vi "LVIS_Test.vi"(8 "Error In":errorcluster, 11 "TestInfo":T1) -> (0 "Error Out":errorcluster)   [LabVIEW 2015]
doc: "Determines the Test Info based on the LVIS_Settings file and passed in values, giving precedence to the file and deriving values where requested. Validates all test data."
uses:
  Sub VIs/Globals/LVIS_IsGlobal.vi
panel:
  out "DateTime":string
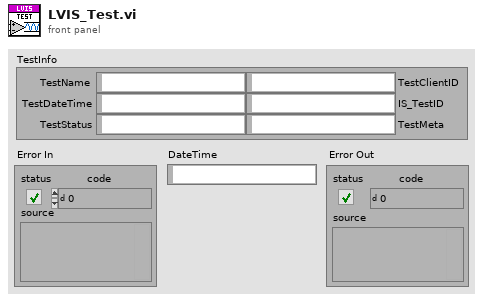
[diagram p1: front panel]
types:
  T1 = cluster{"TestName":string, "TestDateTime":string, "TestStatus":string, "TestClientID":string, "IS_TestID":string, "TestMeta":string}
  T2 = cluster{"[0]":string, "[1]":string, "[2]":string, "[3]":string, "[4]":string, "[5]":string}
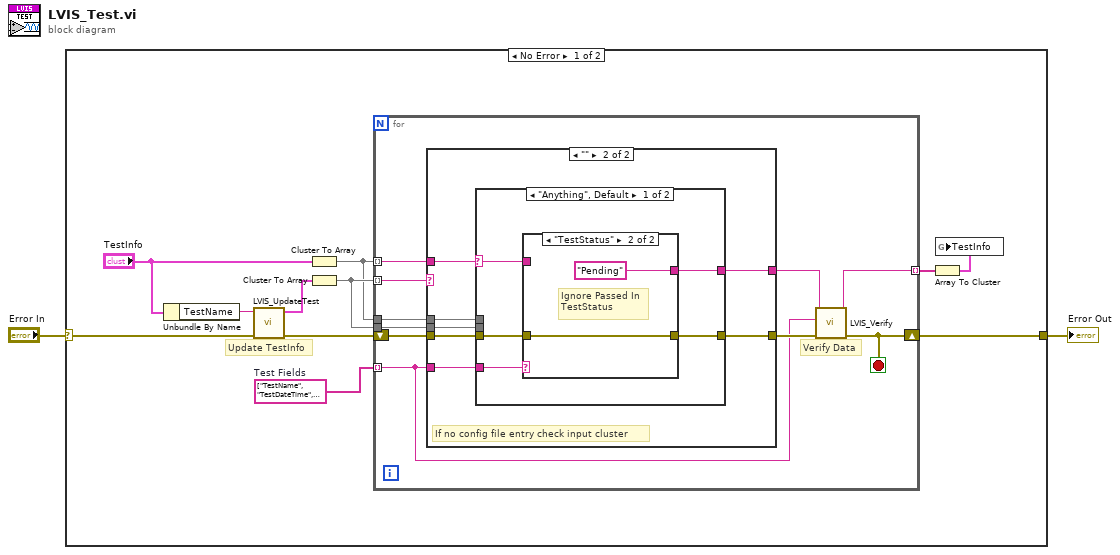
[diagram p0: block diagram]
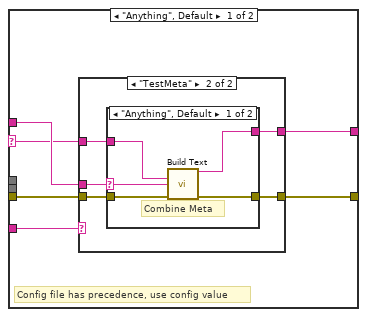
[diagram p2: hidden frame]
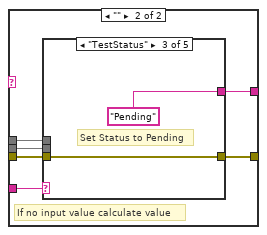
[diagram p6: hidden frame]
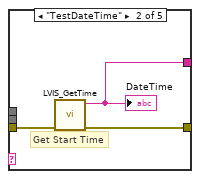
[diagram p8: hidden frame]
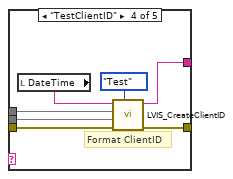
[diagram p9: hidden frame]
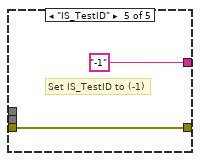
[diagram p10: hidden frame]
diagram:
  n1 = case shown="No Error" "Error In" {
    selector: "Error In" -> [w12 w81]
    tunnel: [w13 w81] -> w2
    frame No Error {
      w11 = string[] ["TestName", "TestDateTime", "TestStatus", "TestClientID", "IS_TestID", "TestMeta"]  # Test Fields
      # "Update TestInfo"
      n2 = Unbundle By Name("TestInfo") -> ("TestName"=w5:string)
      n3 = call "LVIS_UpdateTest.vi"("Error In"=w12, "TestName"=w5) -> ("Error out"=w8:errorcluster, "TestInfo"=w7:T1)  [unwired: 8 in]
      n4 = Cluster To Array(cluster="TestInfo") -> (array=w3:string[])
      n5 = Cluster To Array(cluster=w7) -> (array=w4:string[])
      n6 = for {
        tunnel: w4 -> [w18] mode=indexing
        tunnel: w11 -> [w16] mode=indexing
        shift-right: [w21] -> w13
        shift-left: w8 -> [w23]
        tunnel: w3 -> [w17] mode=indexing
        tunnel: [w19] -> w10 mode=indexing
        tunnel: w4 -> [w15]
        tunnel: w3 -> [w14]
        stop <- w21 stop-if-true
        # "Verify Data"
        n7 = case shown="\"\"" w18 {
          selector: w18 -> [w24 _]
          tunnel: w23 -> [w28 w49]
          tunnel: [w27 w48] -> w22
          tunnel: [w25 w47] -> w20
          tunnel: w16 -> [w29 w46]
          tunnel: w17 -> [w26 w50]
          tunnel: w15 -> [_ w45]
          tunnel: w14 -> [_ w44]
          frame "Anything", Default {
            # "Config file has precedence, use config value"
            n8 = case shown="\"TestMeta\"" w29 {
              tunnel: w28 -> [w31 w36]
              tunnel: [w31 w35] -> w27
              tunnel: w26 -> [_ w33]
              tunnel: [w30 w34] -> w25
              tunnel: w24 -> [w30 w32]
              frame "Other", Default {
                # "Non-Meta Config Data"
              }
              frame "TestMeta" {
                n9 = case shown="\"Anything\", Default" w33 {
                  selector: w33 -> [w37 _]
                  tunnel: w36 -> [w41 w42]
                  tunnel: [w40 w42] -> w35
                  tunnel: [w39 w43] -> w34
                  tunnel: w32 -> [w38 w43]
                  frame "Anything", Default {
                    # "Combine Meta"
                    n10 = call "Build Text"("Meta1"=w38, "Meta2"=w37, "error in (no error)"=w41) -> ("Result"=w39:string, "error out"=w40:errorcluster)  [unwired: 11 in]
                  }
                  frame "" {
                    # "No passed in Meta"
                  }
                }
              }
            }
          }
          frame "" {
            # "If no config file entry check input cluster"
            n11 = case shown="\"Anything\", Default" w50 {
              selector: w50 -> [w53 _]
              tunnel: w49 -> [w55 w65]
              tunnel: [w51 w63] -> w48
              tunnel: [w52 w62] -> w47
              tunnel: w46 -> [w54 w64]
              tunnel: w45 -> [_ w61]
              tunnel: w44 -> [_ w60]
              frame "Anything", Default {
                n12 = case shown="\"TestStatus\"" w54 {
                  tunnel: w55 -> [w56 w58]
                  tunnel: w53 -> [w57 _]
                  tunnel: [w57 "Pending"] -> w52
                  tunnel: [w56 w58] -> w51
                  frame "Anything", Default {
                    # "Use input cluster value"
                  }
                  frame "TestStatus" {
                    # "Ignore Passed In\nTestStatus"
                  }
                }
              }
              frame "" {
                # "If no input value calculate value"
                n13 = case shown="\"TestStatus\"" w64 {
                  tunnel: w65 -> [w66 w69 w71 w78 w79]
                  tunnel: [w66 w68 w71 w77 w79] -> w63
                  tunnel: [_ w67 "Pending" ("Result") w75 "-1" ("ClientID")] -> w62
                  tunnel: w61 -> [_ _ _ w74 _]
                  tunnel: w60 -> [_ _ _ w73 _]
                  frame "Other", Default {
                    # "Value is not calculated"
                  }
                  frame "TestDateTime" {
                    # "Get Start Time"
                    n14 = call "LVIS_GetTime.vi"("Error In"=w69) -> ("Error out"=w68:errorcluster, "DateTime"=w67:string)  [unwired: 9 in]
                    "DateTime" <- w67
                  }
                  frame "TestStatus" {
                    # "Set Status to Pending"
                  }
                  frame "TestClientID" {
                    # "Format ClientID"
                    n15 = local read "DateTime"() -> (w76:string)
                    n16 = call "LVIS_CreateClientID.vi"("Type"=enum16{"Event", "Test", "Meas"}."Test", "Error In"=w78, "CfgInfo"=w74, "InputInfo"=w73, "DateTime"=w76) -> ("Error out"=w77:errorcluster, "ClientID"=w75:string)  [unwired: 5 in]
                  }
                  frame "IS_TestID" {
                    # "Set IS_TestID to (-1)"
                  }
                }
              }
            }
          }
        }
        n17 = call "LVIS_Verify.vi"("Error In"=w22, "Field Name"=w16, "Field Value In"=w20) -> ("Error Out"=w21:errorcluster, "Field Value Out"=w19:string)  [unwired: 7 in]
      }
      n18 = Array To Cluster(array=w10) -> (cluster=w9:T2)
      n19 = global write "LVIS_IsGlobal.vi" "TestInfo"(w9) -> ()
    }
    frame Error {
    }
  }
  "Error Out" <- w2
